vi "Read Info.vi"(8 "error in (no error)":errorcluster, 11 "FormulaG API in":refnum<class "FormulaG API.lvclass">) -> (0 "error out":errorcluster, 2 "Info":T1, 3 "FormulaG API out":refnum<class "FormulaG API.lvclass">)   [LabVIEW 2020, in "FormulaG.lvlib" / "FormulaG API.lvclass"]
uses:
  FormulaG API.lvclass
  FormulaLV-Common/Car Info.ctl
  Command.ctl
  FormulaG API.lvclass/FormulaG API.ctl
  <vilib>/IlluminatedG/lv-stream/stream/Stream.lvclass/Stream.ctl
  <vilib>/IlluminatedG/lv-stream/stream/Dispatch Sniffer Data.vi
  <vilib>/IlluminatedG/lv-stream/stream/Prepared.vi
  <vilib>/IlluminatedG/lv-stream/Endpoint/Cast Sniffer Callback.vi
  <vilib>/IlluminatedG/IG WebSocket Stream/Stream-Websocket/WebsocketStream/WebsocketStream.lvclass
  C:/Program Files (x86)/National Instruments/LabVIEW 2020/vi.lib/IlluminatedG/lv-stream/stream/Stream.lvclass
  <vilib>/Utility/error.llb/Error Cluster From Error Code.vi
  <vilib>/IlluminatedG/lv-stream/stream/Stream.lvclass
  FormulaLV-Common/FormulaG-Common.lvlib
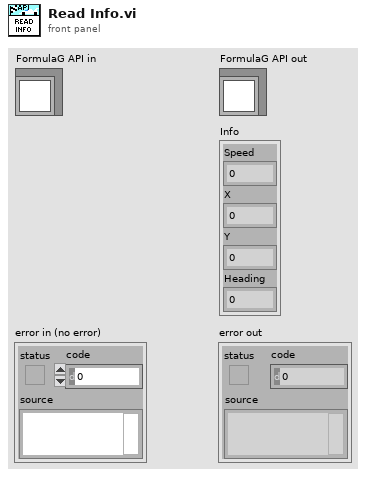
[diagram p1: front panel]
types:
  T1 = typedef "FormulaG-Common.lvlib/Car Info.ctl" = cluster{"Speed":sgl, "X":sgl, "Y":sgl, "Heading":sgl}
  T2 = enum16{"big-endian, network order", "native, host order", "little-endian"}
  T3 = typedef "FormulaG.lvlib/FormulaG API.lvclass/Command.ctl" = enum8{"None", "Reset Car", "Request Ranges", "Control Car", "Request Info", "Set Options", "Set Camera", "Set Pause", "Request Time"}
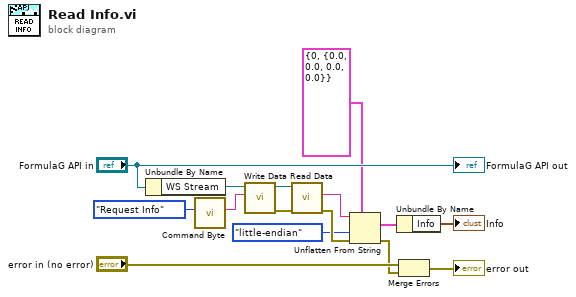
[diagram p0: block diagram]
diagram:
  n1 = Unbundle By Name("FormulaG API in") -> ("WS Stream"=w8:refnum<class "WebsocketStream.lvclass">)
  n2 = call "Command Byte.vi"("Command"=Command."Request Info") -> ("Command Byte"=w7:string)  [unwired: 10 in]
  n3 = call <vilib>:"Write Data.vi"("Data"=w7, "Stream in"=w8) -> ("error out"=w6:errorcluster, "Stream out"=w11:refnum<class "WebsocketStream.lvclass">)  [unwired: 8 in]
  n4 = call <vilib>:"Read Data.vi"("error in (no error)"=w6, "Stream in"=w11) -> ("error out"=w15:errorcluster, "Data"=w10:string)  [unwired: 7 in, 1 out]
  n5 = Unflatten From String(type=cluster{"ID":u8, "Info":T1} {"ID"=0, "Info"={"Speed"=0.0, "X"=0.0, "Y"=0.0, "Heading"=0.0}}, binary string=w10, byte order (0:big-endian, network order)=T2."little-endian", error in (no error)=w15) -> (value=w4:cluster{"ID":u8, "Info":T1}, error out=w1:errorcluster)  [unwired: 1 in, 1 out]
  n6 = Unbundle By Name(w4) -> ("Info"=→"Info":T1)
  n7 = Merge Errors("error in (no error)", w1) -> (→"error out":errorcluster)
  "FormulaG API out" <- "FormulaG API in"
